vi "rampup.vi"(6 "# of Samples":sgl=10.0, 10 "Right Power In":i8=100, 11 "Left Power In":i8=100) -> (2 "Right Power Out":i8, 3 "Left Power out":i8)   [LabVIEW 2012, in "BlockParty4150.lvrbt"]
uses:
  BlockParty4150.lvrbt
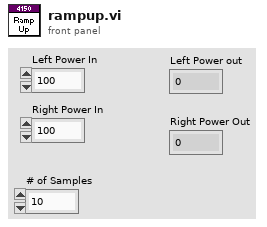
[diagram p1: front panel]
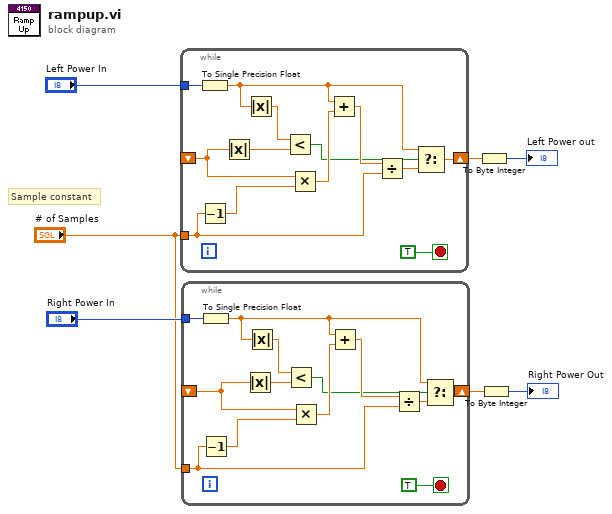
[diagram p0: block diagram]
diagram:
  # "Sample constant"
  n1 = while {
    tunnel: "# of Samples" -> [w15]
    tunnel: "Left Power In" -> [w18]
    shift-right: [w11] -> w6
    shift-left: _ -> [w13]
    stop <- TRUE stop-if-true
    n2 = To Single Precision Float(number=w18) -> (single precision float=w9:sgl)
    n3 = Decrement(x=w15) -> (x-1=w19:sgl)
    n4 = Absolute Value(x=w13) -> (abs(x)=w8:sgl)
    n5 = Absolute Value(x=w9) -> (abs(x)=w14:sgl)
    n6 = Less?(x=w14, y=w8) -> (x < y?=w12:bool)
    n7 = Multiply(x=w13, y=w19) -> (x*y=w17:sgl)
    n8 = Add(x=w9, y=w17) -> (x+y=w16:sgl)
    n9 = Divide(x=w16, y=w15) -> (x/y=w10:sgl)
    n10 = Select(t=w9, s=w12, f=w10) -> (s? t:f=w11:sgl)
  }
  n11 = while {
    tunnel: "# of Samples" -> [w28]
    tunnel: "Right Power In" -> [w31]
    shift-right: [w24] -> w2
    shift-left: _ -> [w26]
    stop <- TRUE stop-if-true
    n12 = To Single Precision Float(number=w31) -> (single precision float=w22:sgl)
    n13 = Decrement(x=w28) -> (x-1=w32:sgl)
    n14 = Absolute Value(x=w26) -> (abs(x)=w21:sgl)
    n15 = Absolute Value(x=w22) -> (abs(x)=w27:sgl)
    n16 = Less?(x=w27, y=w21) -> (x < y?=w25:bool)
    n17 = Multiply(x=w26, y=w32) -> (x*y=w30:sgl)
    n18 = Add(x=w22, y=w30) -> (x+y=w29:sgl)
    n19 = Divide(x=w29, y=w28) -> (x/y=w23:sgl)
    n20 = Select(t=w22, s=w25, f=w23) -> (s? t:f=w24:sgl)
  }
  n21 = To Byte Integer(number=w6) -> (8bit integer=→"Left Power out":i8)
  n22 = To Byte Integer(number=w2) -> (8bit integer=→"Right Power Out":i8)
